vi "Light Panel.vi"() -> ()   [LabVIEW 2014]
uses:
  <vilib>/Platform/TimedLoop/XDataNode/timing_clust.ctl
  <vilib>/Platform/TimedLoop/XDataNode/nitl_modes.ctl
  <vilib>/Platform/TimedLoop/XDataNode/wakeup.ctl
  <vilib>/Platform/TimedLoop/XDataNode/XDataNode.xnode
  <vilib>/Platform/TimedLoop/XDataNode/XDNodeRunTimeDep.lvlib
panel:
  in  "HMI SAFETY CONTROL":bool
  in  "INTENSITY 3":i32(knob) scale=0.0..127.0
  in  "HMI2 Lock":u8
  in  "HMI1 Lock":u8
  in  "TCPConRef":refnum<k5>
  in  "HMI 2":bool
  in  "HMI 1":bool
  in  "Light 4":bool
  in  "Light 2":bool
  in  "Light 3":bool
  in  "Light 1":bool
  in  "INTENSITY 2":i32(knob) scale=0.0..127.0
  in  "INTENSITY 1":i32(knob) scale=0.0..127.0
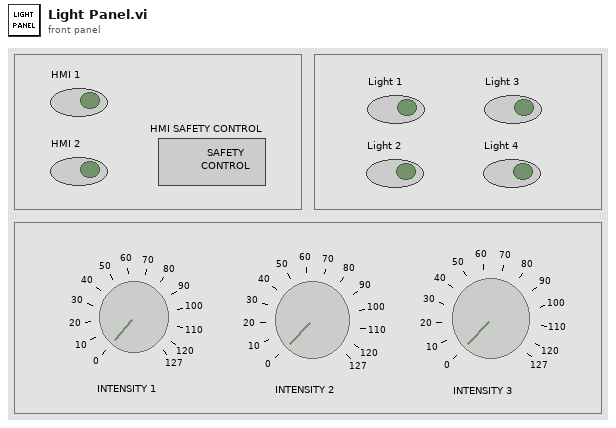
[diagram p1: front panel]
types:
  T1 = typedef "XDNodeRunTimeDep.lvlib/timing_clust.ctl" = cluster{"Expected End [f-1]":u64, "Actual End [f-1]":u64, "Finished Late? [f-1]":bool, "Expected End [i-1]":u64, "Actual End [i-1]":u64, "Finished Late? [i-1]":bool, "Expected Start [i]":u64, "Actual Start [i]":u64, "Expected Start [f]":u64, "Actual Start [f]":u64, "Source Name":string, "Structure Name":string, "Period":i64, "Deadline":i64, "Offset":i64, "Start":i64, "Priority":i32, "Timeout":i32, "Mode":T2, "Wakeup Reason":T3, "Error":errorcluster, "Source Type":string, "Secondary Source Type":string, "Global End Time":u64, "Global Start Time":u64, "Frame Duration":u64, "Iteration Duration":u64, "Assigned CPU":i32, "I/O Scan Engine Mode":u32}
  T2 = typedef "XDNodeRunTimeDep.lvlib/nitl_modes.ctl" = enum32{"No Change", "Process missed periods, maintain original phase", "Discard missed periods, maintain original phase", "Process missed periods, ignore original phase", "Discard missed periods, ignore original phase"}
  T3 = typedef "XDNodeRunTimeDep.lvlib/wakeup.ctl" = enum32{"Normal", "Aborted", "Asynchronous wakeup", "Timing source error", "Timed loop error", "Timeout"}
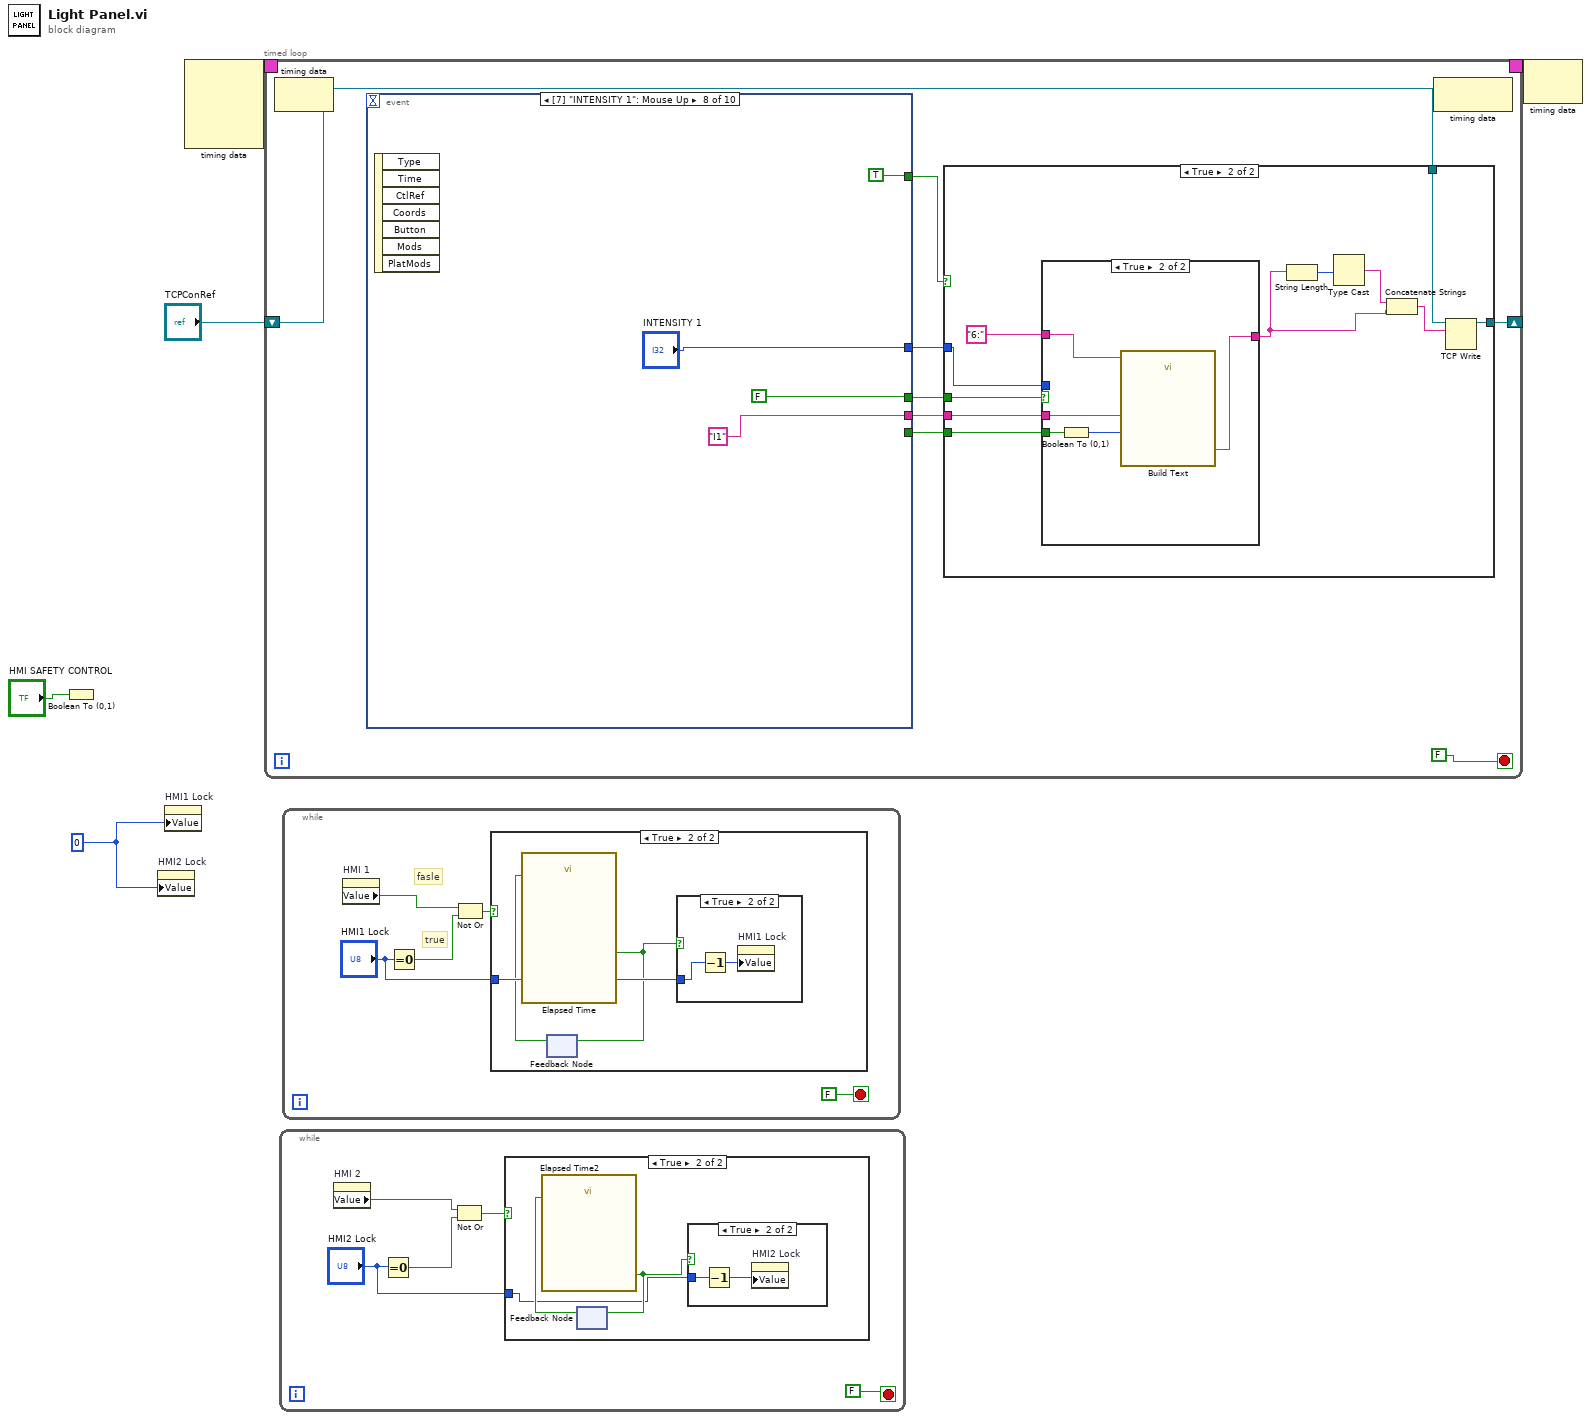
[diagram p0: block diagram]
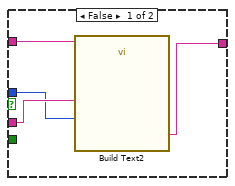
[diagram p3: hidden frame]
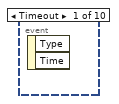
[diagram p4: hidden frame]
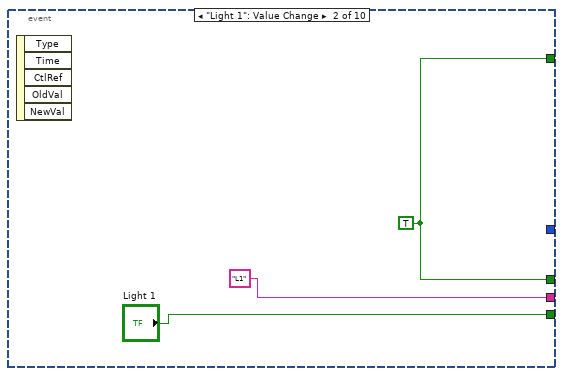
[diagram p5: hidden frame]
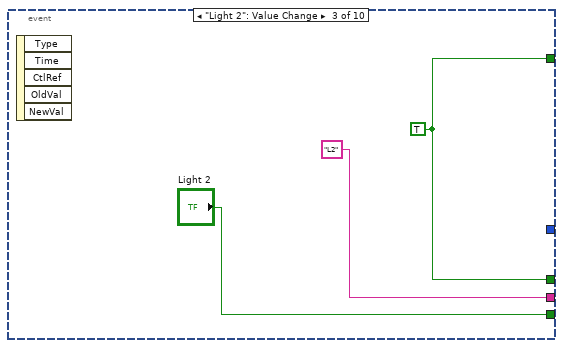
[diagram p6: hidden frame]
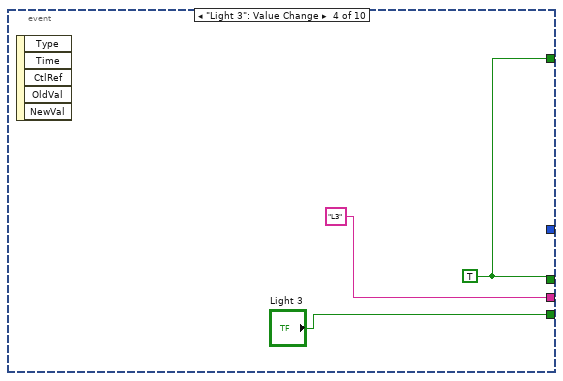
[diagram p7: hidden frame]
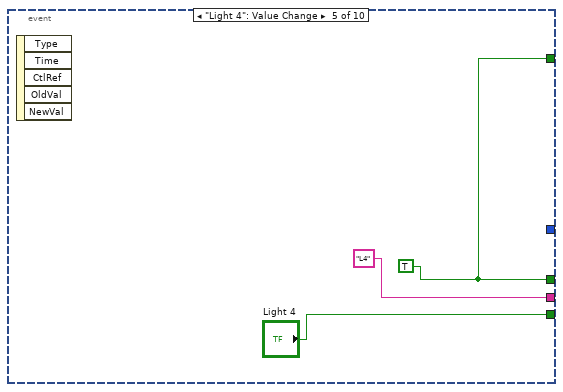
[diagram p8: hidden frame]
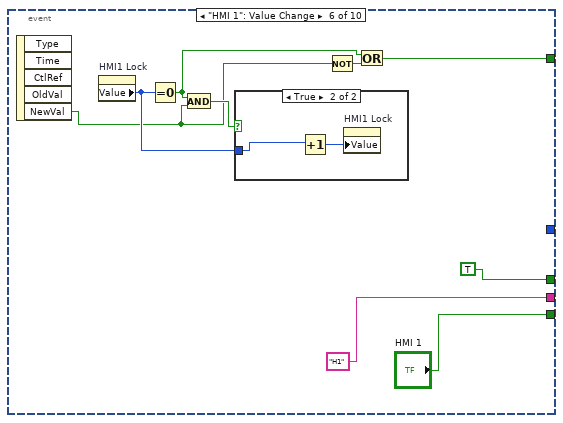
[diagram p9: hidden frame]
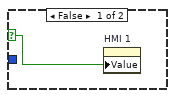
[diagram p10: hidden frame]
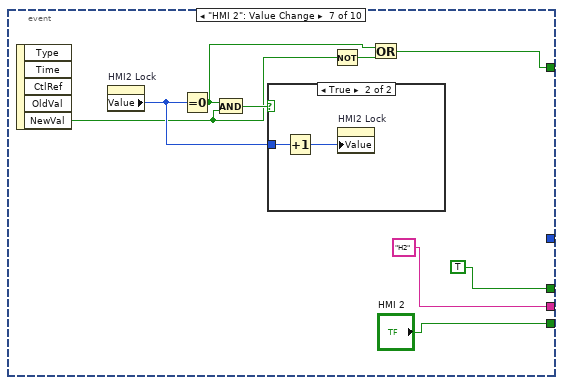
[diagram p11: hidden frame]
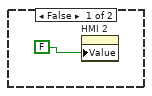
[diagram p12: hidden frame]
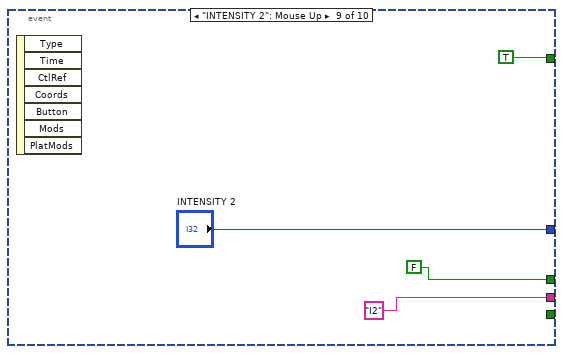
[diagram p13: hidden frame]
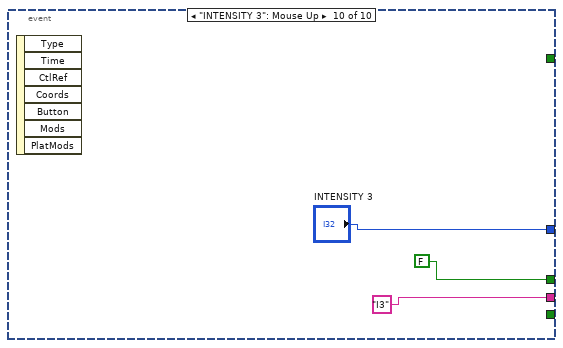
[diagram p14: hidden frame]
diagram:
  w1 = u8 0 ("HMI1 Lock")
  n1 = Boolean To (0,1)(Boolean="HMI SAFETY CONTROL") -> ()  [unwired: 1 out]
  n2 = property on="HMI2 Lock" class="DigNum (strict)"("Value"=w1) -> ()  [unwired: 2 in, 2 out]
  n3 = property on="HMI1 Lock" class="DigNum (strict)"("Value"=w1) -> ()  [unwired: 2 in, 2 out]
  n4 = node-c288() -> (w4:T1)  [unwired: 4 in]
  n5 = timed-loop {
    shift-right: [w7] -> _
    shift-left: "TCPConRef" -> [w8]
    timing: w4 -> [_]
    timing-out: [_] -> w3
    stop <- FALSE stop-if-true
    n6 = node-c288() -> ()  [unwired: 1 in, 1 out]
    n7 = event shown="[7] \"INTENSITY 1\": Mouse Up" {
      selector: _ -> [_ _ _ _ _ _ _ _ _ _]
      dyn-events: _ -> [_ _ _ _ _ _ _ _ _ _]
      timeout: _ -> [_ _ _ _ _ _ _ _ _ _]
      tunnel: [_ "Light 1" "Light 2" "Light 3" "Light 4" "HMI 1" "HMI 2" _ _ _] -> w12
      tunnel: [_ "L1" "L2" "L3" "L4" "H1" "H2" "I1" "I2" "I3"] -> w11
      tunnel: [_ w37 w40 w43 w46 TRUE TRUE FALSE FALSE FALSE] -> w10
      tunnel: [_ _ _ _ _ _ _ "INTENSITY 1" "INTENSITY 2" "INTENSITY 3"] -> w9
      tunnel: [_ w37 w40 w43 w46 w52 w61 TRUE TRUE _] -> w6
      event Timeout {
        n8 = event-data() -> ()  [unwired: 1 in, 2 out]
      }
      event "Light 1": Value Change {
        w37 = TRUE
        n9 = event-data() -> ()  [unwired: 1 in, 5 out]
      }
      event "Light 2": Value Change {
        w40 = TRUE
        n10 = event-data() -> ()  [unwired: 1 in, 5 out]
      }
      event "Light 3": Value Change {
        w43 = TRUE
        n11 = event-data() -> ()  [unwired: 1 in, 5 out]
      }
      event "Light 4": Value Change {
        w46 = TRUE
        n12 = event-data() -> ()  [unwired: 1 in, 5 out]
      }
      event "HMI 1": Value Change {
        n13 = event-data() -> ("NewVal"=w54:bool)  [unwired: 1 in, 4 out]
        n14 = property on="HMI1 Lock" class="DigNum (strict)"() -> ("Value"=w56:u8)  [unwired: 2 in, 2 out]
        n15 = Equal To 0?(x=w56) -> (x = 0?=w53:bool)
        n16 = And(x=w53, y=w54) -> (x .and. y?=w57:bool)
        n17 = case shown="True" w57 {
          selector: w57 -> [w58 _]
          tunnel: w56 -> [_ w59]
          frame False {
            n18 = property on="HMI 1" class="Bool (strict)"("Value"=w58) -> ()  [unwired: 2 in, 2 out]
          }
          frame True {
            n19 = Increment(x=w59) -> (x+1=w60:u8)
            n20 = property on="HMI1 Lock" class="DigNum (strict)"("Value"=w60) -> ()  [unwired: 2 in, 2 out]
          }
        }
        n21 = Not(x=w54) -> (.not. x?=w55:bool)
        n22 = Or(x=w53, y=w55) -> (x .or. y?=w52:bool)
      }
      event "HMI 2": Value Change {
        n23 = event-data() -> ("NewVal"=w62:bool)  [unwired: 1 in, 4 out]
        n24 = property on="HMI2 Lock" class="DigNum (strict)"() -> ("Value"=w65:u8)  [unwired: 2 in, 2 out]
        n25 = Equal To 0?(x=w65) -> (x = 0?=w63:bool)
        n26 = And(x=w63, y=w62) -> (x .and. y?=w66:bool)
        n27 = case shown="True" w66 {
          tunnel: w65 -> [_ w72]
          frame False {
            n28 = property on="HMI 2" class="Bool (strict)"("Value"=FALSE) -> ()  [unwired: 2 in, 2 out]
          }
          frame True {
            n29 = Increment(x=w72) -> (x+1=w71:u8)
            n30 = property on="HMI2 Lock" class="DigNum (strict)"("Value"=w71) -> ()  [unwired: 2 in, 2 out]
          }
        }
        n31 = Not(x=w62) -> (.not. x?=w64:bool)
        n32 = Or(x=w63, y=w64) -> (x .or. y?=w61:bool)
      }
      event "INTENSITY 1": Mouse Up {
        n33 = event-data() -> ()  [unwired: 1 in, 7 out]
      }
      event "INTENSITY 2": Mouse Up {
        n34 = event-data() -> ()  [unwired: 1 in, 7 out]
      }
      event "INTENSITY 3": Mouse Up {
        n35 = event-data() -> ()  [unwired: 1 in, 7 out]
      }
    }
    n36 = case shown="True" w6 {
      tunnel: w12 -> [_ w27]
      tunnel: w11 -> [_ w26]
      tunnel: w10 -> [_ w24]
      tunnel: w9 -> [_ w23]
      tunnel: w8 -> [w16 w22]
      tunnel: [w16 w21] -> w7
      frame False {
      }
      frame True {
        n37 = case shown="True" w24 {
          tunnel: w27 -> [_ w33]
          tunnel: w26 -> [w31 w36]
          tunnel: "6:" -> [w30 w35]
          tunnel: [w29 w34] -> w18
          tunnel: w23 -> [w28 _]
          frame False {
            n38 = call "Build Text2"("Beginning Text"=w30, "ControlID"=w31, "ControlValue"=w28) -> ("Result"=w29:string)  [unwired: 11 in, 1 out]
          }
          frame True {
            n39 = Boolean To (0,1)(Boolean=w33) -> (0, 1=w32:i16)
            n40 = call "Build Text"("Beginning Text"=w35, "ControlID"=w36, "ControlValue"=w32) -> ("Result"=w34:string)  [unwired: 11 in, 1 out]
          }
        }
        n41 = String Length(string=w18) -> (length=w20:i32)
        n42 = Type Cast(x=w20) -> (*(type *) &x=w19:string)  [unwired: 1 in]
        n43 = Concatenate Strings(w19, w18) -> (w17:string)
        n44 = TCP Write(connection ID=w22, data in=w17) -> (connection ID out=w21:refnum<k5>)  [unwired: 2 in, 2 out]
      }
    }
    n45 = node-c288() -> ()  [unwired: 1 in, 1 out]
  }
  n46 = while {
    stop <- FALSE stop-if-true
    n47 = property on="HMI 2" class="Bool (strict)"() -> ("Value"=w87:bool)  [unwired: 2 in, 2 out]
    n48 = Equal To 0?(x="HMI2 Lock") -> (x = 0?=w88:bool)
    n49 = Not Or(1:w88, 2:w87) -> (0:w84:bool)
    n50 = case shown="True" w84 {
      tunnel: "HMI2 Lock" -> [_ w89]
      frame False {
      }
      frame True {
        n51 = feedback #1() -> (w91:bool)  [unwired: 1 in]
        n52 = call "Elapsed Time2"("Reset"=w91) -> ("Time has Elapsed"=w90:bool)  [unwired: 11 in, 7 out]
        n53 = feedback-in #1(w90) -> ()
        n54 = case shown="True" w90 {
          tunnel: w89 -> [_ w93]
          frame False {
          }
          frame True {
            n55 = Decrement(x=w93) -> (x-1=w92:u8)
            n56 = property on="HMI2 Lock" class="DigNum (strict)"("Value"=w92) -> ()  [unwired: 2 in, 2 out]
          }
        }
      }
    }
  }
  n57 = while {
    stop <- FALSE stop-if-true
    # "true"
    # "fasle"
    n58 = property on="HMI 1" class="Bool (strict)"() -> ("Value"=w95:bool)  [unwired: 2 in, 2 out]
    n59 = Equal To 0?(x="HMI1 Lock") -> (x = 0?=w97:bool)
    n60 = Not Or(1:w97, 2:w95) -> (0:w94:bool)
    n61 = case shown="True" w94 {
      tunnel: "HMI1 Lock" -> [_ w101]
      frame False {
      }
      frame True {
        n62 = feedback #2() -> (w99:bool)  [unwired: 1 in]
        n63 = call "Elapsed Time"("Reset"=w99) -> ("Time has Elapsed"=w100:bool)  [unwired: 11 in, 7 out]
        n64 = feedback-in #2(w100) -> ()
        n65 = case shown="True" w100 {
          tunnel: w101 -> [_ w102]
          frame False {
          }
          frame True {
            n66 = Decrement(x=w102) -> (x-1=w103:u8)
            n67 = property on="HMI1 Lock" class="DigNum (strict)"("Value"=w103) -> ()  [unwired: 2 in, 2 out]
          }
        }
      }
    }
  }
  n68 = node-c288(w3) -> ()  [unwired: 1 out]
